vi "InterceptBall.vi"(4 "vf":dbl, 5 "target":dbl[](array[numeric]), 6 "vi":dbl, 7 "firstCall":bool, 8 "error in (no error)":errorcluster, 9 "Robot":refnum<class "Robot.lvclass">, 10 "Game":refnum<class "Game.lvclass">, 11 "WaitBallTrajSkill in":refnum<class "WaitBallTrajSkill.lvclass">) -> (0 "error out":errorcluster, 2 "robot out":refnum<class "Robot.lvclass">, 3 "WaitBallTrajSkill out":refnum<class "WaitBallTrajSkill.lvclass">)   [LabVIEW 2024, in "WaitBallTrajSkill.lvclass"]
uses:
  WaitBallTrajSkill.lvclass
  Game_class/Game.lvclass
  Robot_class/Robot.lvclass
  C:/Users/moise/Documents/GitHub/SSL_AI/Object_class/Object.lvclass
  Robot_class/robotKickToStates.ctl
  Object_class/Object.lvclass/Object.ctl
  Game_class/Game.lvclass/Game.ctl
  Parameters_class/Parameters.lvclass/Parameters.ctl
  Ball_class/Ball.lvclass/Ball.ctl
  Field_class/Field.lvclass/Field.ctl
  Robot_class/Robot.lvclass/Robot.ctl
  <vilib>/Analysis/baseanly.llb/Unit Vector (DBL).vi
  Parameters_class/Read KickForce.vi
  Game_class/Read Parameters.lvclass.vi
  Game_class/Read BallRef.vi
  Game_class/Read FieldRef.vi
  Game_class/Read NewParameters.vi
  Field_class/Read ourGoalPosition.vi
  Field_class/Read enemyGoalPosition.vi
  Object_class/Read position(x,y).vi
  Ball_class/Read velocityNorm.vi
  Ball_class/Read v_x.vi
  Ball_class/Read v_y.vi
  Parameters_class/Read BallVelToAbortPass.vi
  Parameters_class/Read AttakingOurselves.vi
  Robot_class/Write dest_x.vi
  Robot_class/Write dest_y.vi
  Robot_class/Write dest_orientation.vi
  Robot_class/Write dribble.vi
  Robot_class/Write kick_x.vi
  Robot_class/Write keepDest.vi
  Robot_class/Write robotKickState.vi
  <vilib>/Analysis/_algsub.llb/Vector Norm.vi
  <vilib>/Analysis/_algsub.llb/Real Vector Norm.vi
  Ball_class/Ball.lvclass
  Parameters_class/Parameters.lvclass
  Field_class/Field.lvclass
  Utilities_class/Utilities.lvclass
  <vilib>/Analysis/NI_AALBase.lvlib
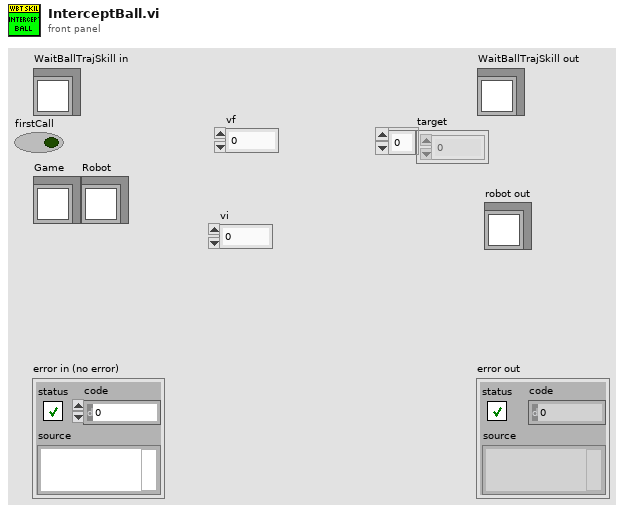
[diagram p1: front panel]
types:
  T1 = typedef "robotKickToStates.ctl" = enum16{"shootFromDirect", "avoidCollideBall", "goToBackBall", "none", "walk", "turn", "turnAntiClockWise", "turnClockwise", "oldKickToShoot", "oldKickToGoToBackBall", "shoot"}
  T2 = typedef "NewParameters.ctl" = cluster{"PenaltyDistance":dbl, "DistanceAttackerToBackBall":dbl, "Division":enum16{"Div B", "Div A"}, "DistanceToAvoidyEnemyRobot":dbl, "BallPlacementDistance":dbl, "DisatanceBehindBallToStealBall":dbl, "MaxDistanceToPositionKickoff":dbl, "BlockEnemyTarget":bool, "MaxStopVAng":dbl, "DistanceMarkerToEnemy":dbl, "IgnoreDribblerContact":bool, "DistanceToBeginEnemyPosession":dbl, "GoToBallWhenEnemyNotMoving":bool, "EnemyDistanceToReduceVelocity":dbl, "TurnOnEnemyDistanceToReduceVelocity":bool, "EnemyDistanceToShootOutBall":dbl, "DefenseKickBall":bool, "MoreKickToGoal? (0-0.3)":dbl, "ChipKickInEnemyField":bool, "ShootOutRobotId":dbl, "FieldLenghtDenominatorInShootOut":dbl, "AdjustPositionInBallPlacement":bool, "PowerGodPass":dbl, "VelocityAbortEnemyPos":dbl, "MaxDistToBeginPass":dbl, "MinDistToBeginPass":dbl, "VelocityInDirects":dbl, "BadDribblerIDs":i32[], "NewKickToDistanceAroundBall":dbl, "PowerAvoidColisionMarker":dbl, "DistanceToAvoidColisionMarker":dbl, "AvoidBallKick":dbl, "DistanceTryKick":dbl, "SuicideKickDIstance":dbl, "AdjustFirstKickDistance":dbl, "AvoidAimLessKick":dbl, "DistanceToAvoidyEnemyShootRobot ":dbl, "NumberOfMarkers":dbl, "PotField":bool, "PIDLateral":bool, "MinDistanceFirstKickX":dbl, "MinDistanceFirstKickY":dbl, "FractionOfDistToTouchGround\nAfterChipKick":dbl, "FractionOfKickxWhen\nComposedWithKickz":dbl, "Style":T3, "MoveInTurnState":bool, "DistFromEnemyToConsider\nMoveInTurnState":dbl, "CascadePID":bool, "TurnAroundParameters":cluster{"Radius":dbl, "Multiplier":dbl, "ChordAngle":dbl}, "SafeDriveVel":dbl, "DistanceToGoToBackBall":dbl, "minDistanceToNotFinish\nEnemyPossession":dbl, "OneTouchShot":cluster{"angleFactor":dbl, "maxAngle":dbl, "Attack":bool, "Defense":bool}, "OpenAngleToGoal":cluster{"minAngle":dbl, "maxAngle":dbl, "minEvaluation":dbl}, "ShotInterception":cluster{"shotSpeed":dbl, "minEnemySpeed":dbl, "maxEnemySpeed":dbl, "minEvaluation":dbl}, "AllyTeamArray":T4[], "maxDefendersNumber":i32, "Zone":cluster{"GuardPositionArray":dbl[][], "ZoneMidField":dbl[], "CenterForwardWidth":dbl}, "MinEvaluationToShoot":dbl, "PassInterception":cluster{"maxPassSpeed":dbl, "minPassSpeed":dbl, "minEnemySpeed":dbl, "chipPassDistance":dbl, "chipPassEvaluation":dbl, "minEvaluation":dbl, "maxEnemySpeed":dbl}, "PassDistance":cluster{"maxDistance":dbl, "minDistance":dbl}, "receiverSpeed":dbl, "maxBallSpeed":dbl, "slackTime":dbl, "Turning radius":dbl, "Turning v_ang":dbl, "AlignError":cluster{"Distance":dbl, "Orientation":dbl, "V_norm(m/s)":dbl, "V_ang (rad/s)":dbl}, "RobotRadius":dbl, "KickerDistance":dbl, "keeper angle  to cover goalpost":dbl, "a_slide":dbl, "a_roll":dbl, "k_switch":dbl}
  T3 = typedef "Style.ctl" = enum16{"Insanity", "Offensive", "Defensive"}
  T4 = typedef "AllyTeam.ctl" = enum16{"Keeper", "Defender", "Attacker"}
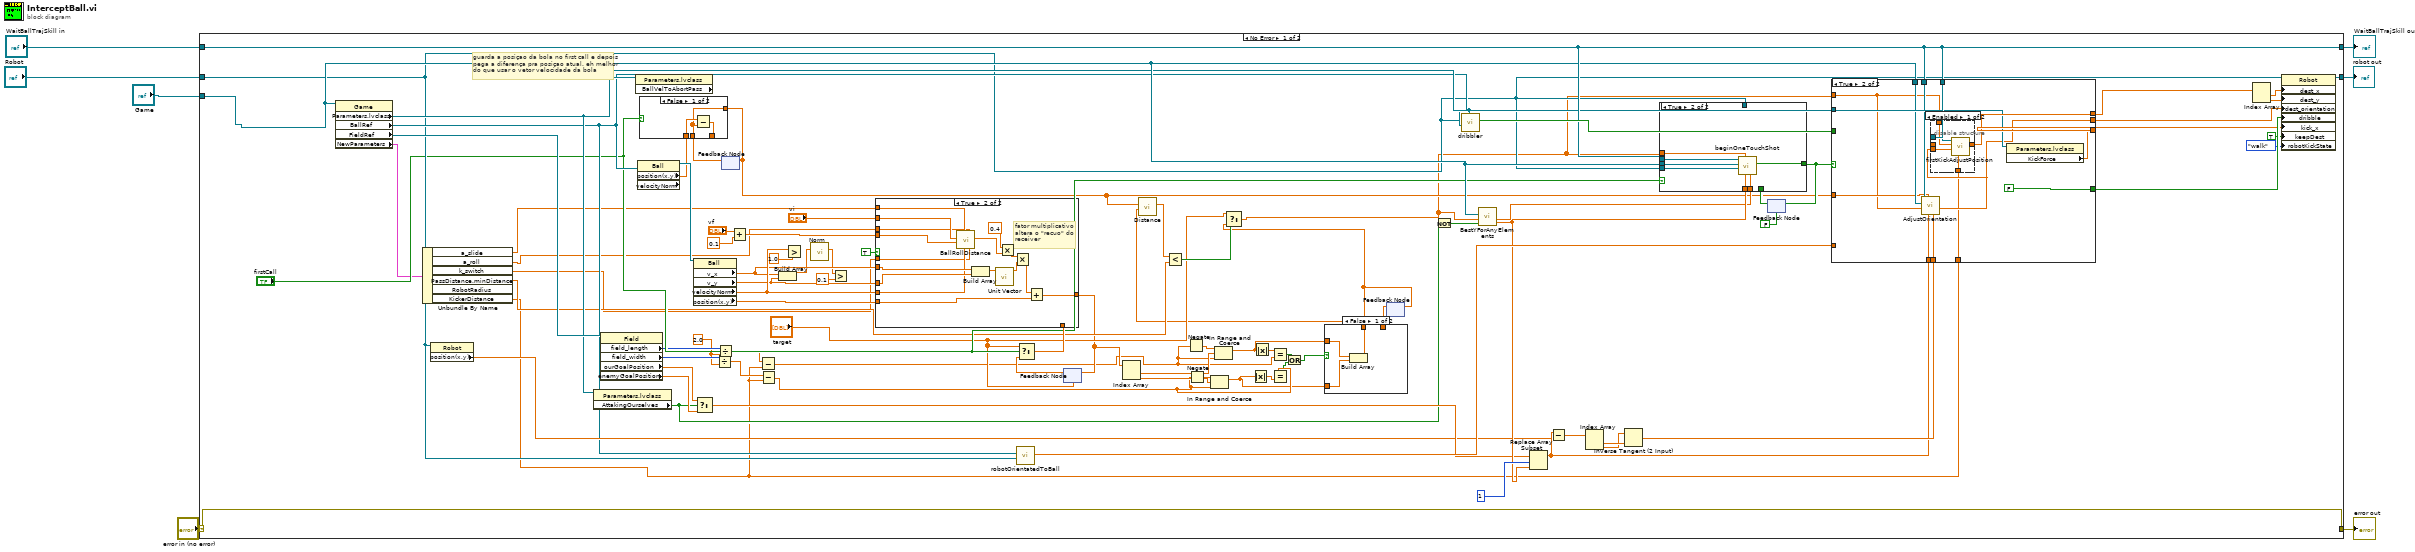
[diagram p0: block diagram]
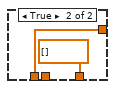
[diagram p4: hidden frame]
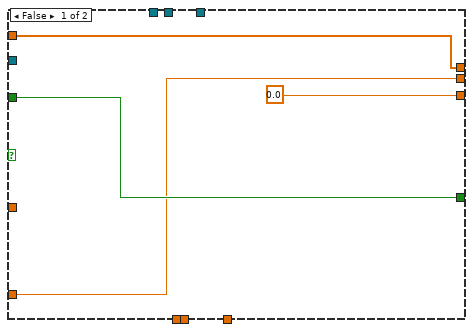
[diagram p6: hidden frame]
diagram:
  n1 = case shown="No Error" "error in (no error)" {
    selector: "error in (no error)" -> [w93 w152]
    tunnel: [w93 w152] -> w6
    tunnel: [w72 w151] -> w4
    tunnel: "WaitBallTrajSkill in" -> [w72 w151]
    tunnel: "Robot" -> [w59 _]
    tunnel: "Game" -> [w71 _]
    tunnel: [w92 _] -> w2
    frame No Error {
      w43 = 2.0 ("y")
      # "guarda a posiçao da bola no first call e depois\npega a diferença pra posiçao atual. eh melhor\ndo que usar o vetor velocidade da bola"
      n2 = property class="Game"(reference=w71) -> ("Parameters.lvclass"=w63:refnum<class "Parameters.lvclass">, "BallRef"=w60:refnum<class "Ball.lvclass">, "FieldRef"=w91:refnum<class "Field.lvclass">, "NewParameters"=w42:T2)  [unwired: 1 in, 2 out]
      n3 = Unbundle By Name(w42) -> ("a_slide"=w23:dbl, "a_roll"=w22:dbl, "k_switch"=w21:dbl, "PassDistance.minDistance"=w29:dbl, "KickerDistance"=w19:dbl)  [unwired: 1 out]
      n4 = property class="Robot"(reference=w59) -> ("position(x,y)"=w62:dbl[])  [unwired: 1 in, 2 out]
      n5 = property class="Parameters.lvclass"(reference=w63) -> ("AttakingOurselves"=w66:bool)  [unwired: 1 in, 2 out]
      n6 = property class="Field"(reference=w91) -> ("field_length"=w45:i32, "field_width"=w44:i32, "ourGoalPosition"=w69:dbl[], "enemyGoalPosition"=w68:dbl[])  [unwired: 1 in, 2 out]
      n7 = property class="Parameters.lvclass" props=["BallVelToAbortPass"](reference=w63) -> ()  [unwired: 1 in, 3 out]
      n8 = property class="Ball" props=["position(x,y)", "velocityNorm"](reference=w60) -> (reference out=w56:refnum<class "Ball.lvclass">, "position(x,y)"=w49:dbl[])  [unwired: 1 in, 2 out]
      n9 = property class="Ball"(reference=w56) -> ("v_x"=w37:dbl, "v_y"=w36:dbl, "velocityNorm"=w55:dbl, "position(x,y)"=w51:dbl[])  [unwired: 1 in, 2 out]
      n10 = Select(t=w69, s=w66, f=w68) -> (s? t:f=w67:dbl[])
      n11 = Divide(x=w44, y=w43) -> (x/y=w40:dbl)
      n12 = Divide(x=w45, y=w43) -> (x/y=w41:dbl)
      n13 = feedback #1() -> (w61:dbl[])  [unwired: 1 in]
      n14 = case shown="False" "firstCall" {
        tunnel: w49 -> [w117 w119]
        tunnel: w61 -> [w116 _]
        tunnel: [w116 w119] -> w31
        tunnel: [w115 dbl[] []] -> _
        frame False {
          n15 = Subtract(x=w117, y=w116) -> (x-y=w115:dbl[])
        }
        frame True {
        }
      }
      n16 = feedback-in #1(w31) -> ()
      n17 = Add(x="vf", y=0.1) -> (x+y=w54:dbl)
      n18 = Subtract(x=w41, y=w19) -> (x-y=w16:dbl)
      n19 = Subtract(x=w40, y=w19) -> (x-y=w15:dbl)
      n20 = Build Array(w37, w36) -> (w35:dbl[])
      n21 = Greater?(x=w55, y=1.0) -> ()  [unwired: 1 out]
      n22 = call "Norm.vi"("2D vector"=w35) -> ("Modulo"=w34:dbl)  [unwired: 8 in, 2 out]
      n23 = Greater?(x=w34, y=0.1) -> ()  [unwired: 1 out]
      n24 = call "robotOrientatedToBall.vi"("Robot"=w59, "BallRef"=w60) -> ("Orientation"=w86:dbl)  [unwired: 7 in, 2 out]
      n25 = feedback #2("target") -> (w52:dbl[])
      n26 = Select(t="target", s="firstCall", f=w52) -> (s? t:f=w53:dbl[])
      n27 = case shown="True" TRUE {
        tunnel: w54 -> [_ w110]
        tunnel: [w98 w109] -> w26
        tunnel: w37 -> [_ w108]
        tunnel: w36 -> [_ w107]
        tunnel: w55 -> [_ w106]
        tunnel: w51 -> [_ w105]
        tunnel: w53 -> [w98 _]
        tunnel: "vi" -> [_ w104]
        tunnel: w23 -> [_ w103]
        tunnel: w22 -> [_ w102]
        tunnel: w21 -> [_ w101]
        frame False {
        }
        frame True {
          # "fator multiplicativo\naltera o \"recuo\" do \nreceiver"
          n28 = call "BallRollDistance.vi"("k_switch"=w101, "acc_roll"=w102, "vcur"=w106, "acc_slide"=w103, "vf"=w110, "vi"=w104) -> ("dist"=w113:dbl)  [unwired: 3 in, 2 out]
          n29 = Build Array(w108, w107) -> (w111:dbl[])
          n30 = call-poly <vilib>:"Unit Vector.vi"("Input Vector"=w111) -> ("Unit Vector"=w112:dbl[])  [unwired: 8 in, 2 out]
          n31 = Multiply(x=0.4, y=w113) -> (x*y=w100:dbl)
          n32 = Multiply(x=w100, y=w112) -> (x*y=w114:dbl[])
          n33 = Add(x=w114, y=w105) -> (x+y=w109:dbl[])
        }
      }
      n34 = feedback-in #2(w26) -> ()
      n35 = Index Array(array=w26) -> (element #1=w48:dbl, element #2=w47:dbl)  [unwired: 2 in]
      n36 = Negate(x=w16) -> (-x=w46:dbl)
      n37 = Negate(x=w15) -> (-x=w39:dbl)
      n38 = In Range and Coerce(upper limit=w39, x=w47, lower limit=w15) -> (coerced(x)=w10:dbl)  [unwired: 1 out]
      n39 = In Range and Coerce(upper limit=w46, x=w48, lower limit=w16) -> (coerced(x)=w11:dbl)  [unwired: 1 out]
      n40 = Absolute Value(x=w10) -> (abs(x)=w17:dbl)
      n41 = Absolute Value(x=w11) -> (abs(x)=w18:dbl)
      n42 = Equal?(x=w18, y=w16) -> (x = y?=w14:bool)
      n43 = Equal?(x=w15, y=w17) -> (x = y?=w13:bool)
      n44 = Or(x=w14, y=w13) -> (x .or. y?=w12:bool)
      n45 = feedback #3() -> (w8:dbl[])  [unwired: 1 in]
      n46 = case shown="False" w12 {
        tunnel: w11 -> [w96 _]
        tunnel: w10 -> [w95 _]
        tunnel: [w94 w97] -> w9
        tunnel: w8 -> [_ w97]
        frame False {
          n47 = Build Array(w96, w95) -> (w94:dbl[])
        }
        frame True {
        }
      }
      n48 = call "Distance.vi"("P1"=w9, "P2"=w31) -> ("Distance"=w30:dbl)  [unwired: 7 in, 2 out]
      n49 = Less?(x=w30, y=w29) -> (x < y?=w28:bool)
      n50 = Select(t="target", s=w28, f=w9) -> (s? t:f=w25:dbl[])
      n51 = feedback-in #3(w9) -> ()
      n52 = Not(x=w66) -> (.not. x?=w65:bool)
      n53 = call "dribbler.vi"("Parameters.lvclass"=w63, "Ball"=w60, "Robot"=w59) -> ("Dribbler?"=w89:bool)  [unwired: 6 in, 2 out]
      n54 = call "BestYForAnyElements.vi"("inimigos"=w65, "Position to be analyzed"=w25, "Game"=w71) -> ("Best y"=w70:dbl, "Gap Coord"=w64:dbl[])  [unwired: 5 in, 2 out]
      n55 = Replace Array Subset(array=w67, new element=w70, index=1) -> (w73:dbl[])
      n56 = Subtract(x=w73, y=w62) -> (x-y=w83:dbl[])
      n57 = Index Array(array=w83) -> (element #1=w85:dbl, element #2=w84:dbl)  [unwired: 2 in]
      n58 = Inverse Tangent (2 Input)(1:w85, 2:w84) -> (0:w74:dbl)
      n59 = feedback #4(FALSE ("Boolean")) -> (w78:bool)
      n60 = case shown="True" "firstCall" {
        tunnel: w72 -> [_ w127]
        tunnel: w71 -> [_ w126]
        tunnel: w59 -> [_ w125]
        tunnel: [w120 w124] -> w79
        tunnel: w78 -> [w120 _]
        tunnel: w59 -> [_ _]
        tunnel: w70 -> [_ w123]
        tunnel: w64 -> [_ w122]
        tunnel: w25 -> [_ w121]
        frame False {
        }
        frame True {
          n61 = call "beginOneTouchShot.vi"("Gap Coord"=w122, "bestY"=w123, "targetPosition"=w121, "Robot"=w125, "Game"=w126, "WaitBallTrajSkill in"=w127) -> ("Boolean"=w124:bool)  [unwired: 3 in, 2 out]
        }
      }
      n62 = feedback-in #4(w79) -> ()
      n63 = case shown="True" w79 {
        tunnel: [w131 FALSE ("Dribbler?")] -> w90
        tunnel: w89 -> [w131 _]
        tunnel: [w130 w135] -> w88
        tunnel: w86 -> [w130 _]
        tunnel: [0.0 ("kick_x") w140] -> w87
        tunnel: w63 -> [_ w141]
        tunnel: w72 -> [_ w143]
        tunnel: [w128 w142] -> w82
        tunnel: w74 -> [_ w139]
        tunnel: w73 -> [_ w138]
        tunnel: w71 -> [_ w137]
        tunnel: w72 -> [_ w136]
        tunnel: w31 -> [_ w134]
        tunnel: w25 -> [w128 w133]
        tunnel: w19 -> [_ w132]
        frame False {
        }
        frame True {
          n64 = call "AdjustOrientation.vi"("orientation"=w139, "target"=w138, "initial pos"=w134, "dest"=w133, "Game"=w137, "WaitBallTrajSkill in"=w136) -> ("orientation out"=w135:dbl)  [unwired: 3 in, 2 out]
          n65 = disable-structure shown="Enabled" {
            disable-tunnel: w143 -> [w149 _]
            disable-tunnel: [w148 w150] -> w142
            disable-tunnel: _ -> [_ w150]
            disable-tunnel: w135 -> [w147 _]
            disable-tunnel: w133 -> [w146 _]
            disable-tunnel: w132 -> [w145 _]
            frame Enabled {
              n66 = call "firstKickAdjustPosition.vi"("Dist"=w145, "Orientation"=w147, "Dest"=w146, "WaitBallTrajSkill in"=w149) -> ("AdjustDest"=w148:dbl[])  [unwired: 5 in, 2 out]
            }
            frame Disabled {
            }
          }
          n67 = property class="Parameters.lvclass"(reference=w141) -> ("KickForce"=w140:dbl)  [unwired: 1 in, 2 out]
        }
      }
      n68 = Index Array(array=w82) -> (element #1=w80:dbl, element #2=w81:dbl)  [unwired: 2 in]
      n69 = property class="Robot"(reference=w59, "dest_x"=w80, "dest_y"=w81, "dest_orientation"=w88, "dribble"=w90, "kick_x"=w87, "keepDest"=TRUE, "robotKickState"=robotKickToStates."walk") -> (reference out=w92:refnum<class "Robot.lvclass">)  [unwired: 1 in, 1 out]
    }
    frame Error {
    }
  }
  "error out" <- w6
  "WaitBallTrajSkill out" <- w4
  "robot out" <- w2
